vi "n set offset.vi"(8 "error in (no error)":errorcluster, 9 "yoffset":i16, 10 "xoffset":i16, 11 "n":u16) -> (0 "error out":errorcluster)   [LabVIEW 2015, in "SCANalone4x64.lvlib"]
doc: "__declspec(dllimport) void __stdcall n_set_offset(unsigned short n, short xoffset, short yoffset);"
uses:
  <userlib>/SCANalone4x64/SCANalone4x64.lvlib
  <userlib>/SCANalone4x64/SCANalone4x64.dll
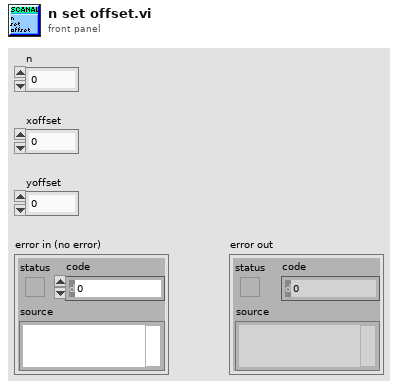
[diagram p1: front panel]
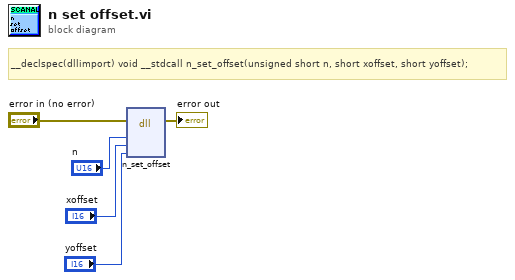
[diagram p0: block diagram]
diagram:
  # "__declspec(dllimport) void __stdcall n_set_offset(unsigned short n, short xoffset, short yoffset);"
  n1 = dll-call lib="C:/Program Files/National Instruments/LabVIEW 2015/user.lib/SCANalone4x64/SCANalone4x64.*" fn="n_set_offset"(error in="error in (no error)", "n"="n", "xoffset"="xoffset", "yoffset"="yoffset") -> (error out=→"error out":errorcluster)  [unwired: 6 in, 1 out]
